vi "map construction.vi"() -> ()   [LabVIEW 2018]
uses:
  <vilib>/vision/NI_Vision_Development_Module.lvlib
panel:
  out "i":i32
  out "Image 7":T1(plugin-control)
  in  "Stop (F)":bool
  out "数值 2":dbl
  out "数值":dbl
  out "数组":sgl[](array[numeric])
  out "Objects":T2(array[cluster]) {"Aspect Ratio" format="%.2f"; "Orientation" format="%.2f"; "Area" format="%.2f"; "Object Center"."Y" format="%.2f"; "Object Center"."X" format="%.2f"}
  in  "Settings":T3={"Objects"=0, "Threshold"=128, "Reject Border"=FALSE, "Fill Holes"=FALSE, "Min Object Size"=TRUE, "Min Size"=5000, "Max Object Size"=FALSE, "Max Size"=100, "Show Search Area"=FALSE, "Show Center"=TRUE, "Show Bounding Box"=TRUE} {"Objects" items=["Bright Objects", "Dark Objects"]; "Threshold" min=1 max=999999999 step=1; "Max Size" min=1 max=999999999 step=1; "Min Size" min=1 max=999999999 step=1}
  out "Image 2":T1(plugin-control)
  in  "Range":cluster{"Lower value":sgl, "Upper value":sgl}={"Lower value"=0.0, "Upper value"=128.0} {"Upper value" format="%.2f"; "Lower value" format="%.2f"}
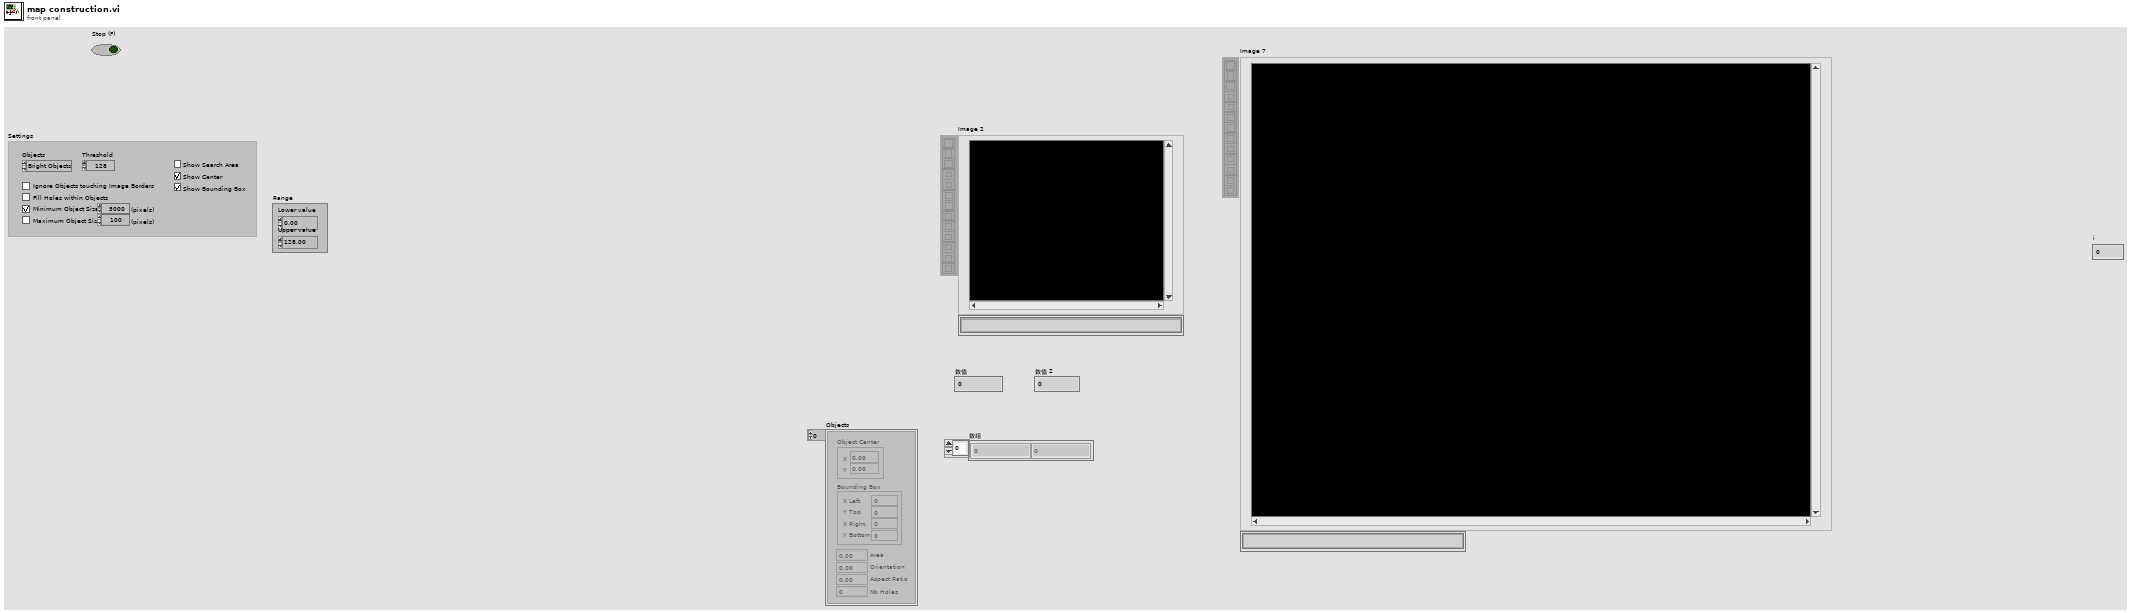
[diagram p1: front panel]
types:
  T1 = typedef "IMAQ Image.ctl" = refnum<image>
  T2 = cluster{"Object Center":cluster{"X":sgl, "Y":sgl}, "Bounding Box":cluster{"X Left":i32, "Y Top":i32, "X Right":i32, "Y Bottom":i32}, "Area":sgl, "Orientation":sgl, "Aspect Ratio":sgl, "Nb Holes":i32}[]
  T3 = cluster{"Objects":u16, "Threshold":i32, "Reject Border":bool, "Fill Holes":bool, "Min Object Size":bool, "Min Size":i32, "Max Object Size":bool, "Max Size":i32, "Show Search Area":bool, "Show Center":bool, "Show Bounding Box":bool}
  T4 = typedef "Image Type" = u32
  T5 = cluster{"Left":i32, "Top":i32, "Right":i32, "Bottom":i32}
  T6 = cluster{"Objects[0]":cluster{"Object Center":cluster{"X":sgl, "Y":sgl}, "Bounding Box":cluster{"X Left":i32, "Y Top":i32, "X Right":i32, "Y Bottom":i32}, "Area":sgl, "Orientation":sgl, "Aspect Ratio":sgl, "Nb Holes":i32}, "Objects[1]":cluster{"Object Center":cluster{"X":sgl, "Y":sgl}, "Bounding Box":cluster{"X Left":i32, "Y Top":i32, "X Right":i32, "Y Bottom":i32}, "Area":sgl, "Orientation":sgl, "Aspect Ratio":sgl, "Nb Holes":i32}, "Objects[2]":cluster{"Object Center":cluster{"X":sgl, "Y":sgl}, "Bounding Box":cluster{"X Left":i32, "Y Top":i32, "X Right":i32, "Y Bottom":i32}, "Area":sgl, "Orientation":sgl, "Aspect Ratio":sgl, "Nb Holes":i32}, "Objects[3]":cluster{"Object Center":cluster{"X":sgl, "Y":sgl}, "Bounding Box":cluster{"X Left":i32, "Y Top":i32, "X Right":i32, "Y Bottom":i32}, "Area":sgl, "Orientation":sgl, "Aspect Ratio":sgl, "Nb Holes":i32}, "Objects[4]":cluster{"Object Center":cluster{"X":sgl, "Y":sgl}, "Bounding Box":cluster{"X Left":i32, "Y Top":i32, "X Right":i32, "Y Bottom":i32}, "Area":sgl, "Orientation":sgl, "Aspect Ratio":sgl, "Nb Holes":i32}, "Objects[5]":cluster{"Object Center":cluster{"X":sgl, "Y":sgl}, "Bounding Box":cluster{"X Left":i32, "Y Top":i32, "X Right":i32, "Y Bottom":i32}, "Area":sgl, "Orientation":sgl, "Aspect Ratio":sgl, "Nb Holes":i32}, "Objects[6]":cluster{"Object Center":cluster{"X":sgl, "Y":sgl}, "Bounding Box":cluster{"X Left":i32, "Y Top":i32, "X Right":i32, "Y Bottom":i32}, "Area":sgl, "Orientation":sgl, "Aspect Ratio":sgl, "Nb Holes":i32}, "Objects[7]":cluster{"Object Center":cluster{"X":sgl, "Y":sgl}, "Bounding Box":cluster{"X Left":i32, "Y Top":i32, "X Right":i32, "Y Bottom":i32}, "Area":sgl, "Orientation":sgl, "Aspect Ratio":sgl, "Nb Holes":i32}, "Objects[8]":cluster{"Object Center":cluster{"X":sgl, "Y":sgl}, "Bounding Box":cluster{"X Left":i32, "Y Top":i32, "X Right":i32, "Y Bottom":i32}, "Area":sgl, "Orientation":sgl, "Aspect Ratio":sgl, "Nb Holes":i32}}
  T7 = cluster{"Object Center":cluster{"X":sgl, "Y":sgl}, "Bounding Box":cluster{"X Left":i32, "Y Top":i32, "X Right":i32, "Y Bottom":i32}, "Area":sgl, "Orientation":sgl, "Aspect Ratio":sgl, "Nb Holes":i32}
  T8 = cluster{"X Left":i32, "Y Top":i32, "X Right":i32, "Y Bottom":i32}
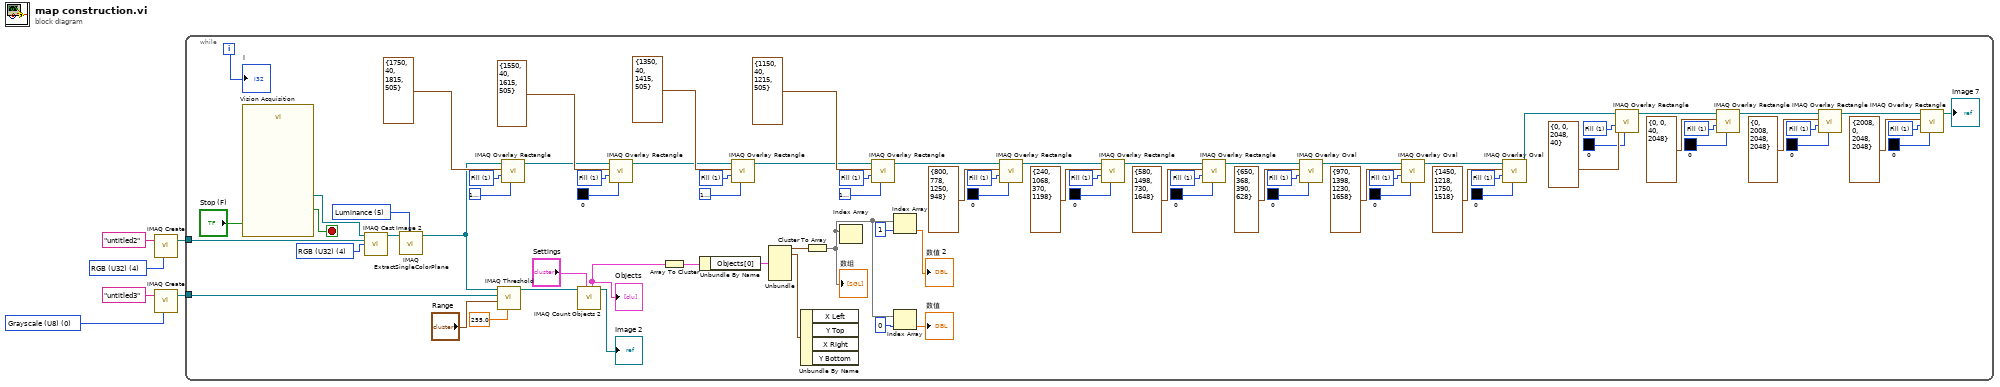
[diagram p0: block diagram]
diagram:
  w1 = T4 0 items=["Grayscale (U8)", "Grayscale (I16)", "Grayscale (SGL)", "Complex (CSG)", "RGB (U32)", "HSL (U32)", "RGB (U64)", "Grayscale (U16)"] ("Image Type")
  w4 = T4 4 items=["Grayscale (U8)", "Grayscale (I16)", "Grayscale (SGL)", "Complex (CSG)", "RGB (U32)", "HSL (U32)", "RGB (U64)", "Grayscale (U16)"] ("Image Type")
  n1 = call "IMAQ Create"("Image Name"="untitled2", "Image Type"=w4) -> ("New Image"=w5:T1)  [unwired: 3 in, 1 out]
  n2 = call "IMAQ Create"("Image Name"="untitled3", "Image Type"=w1) -> ("New Image"=w3:T1)  [unwired: 3 in, 1 out]
  n3 = while {
    tunnel: w5 -> [w87]
    tunnel: w3 -> [w83]
    i -> [w50]
    stop <- w72 stop-if-true
    w8 = u32 1 items=["Frame", "Fill", "Highlight"] ("Drawing Mode (Frame)")
    w11 = u32 1 items=["Frame", "Fill", "Highlight"] ("Drawing Mode (Frame)")
    w14 = u32 1 items=["Frame", "Fill", "Highlight"] ("Drawing Mode (Frame)")
    w17 = u32 1 items=["Frame", "Fill", "Highlight"] ("Drawing Mode (Frame)")
    w25 = u32 1 items=["Frame", "Fill"] ("Drawing Mode (Frame)")
    w28 = u32 1 items=["Frame", "Fill"] ("Drawing Mode (Frame)")
    w33 = u32 1 items=["Frame", "Fill"] ("Drawing Mode (Frame)")
    w46 = u32 1 items=["Frame", "Fill", "Highlight"] ("Drawing Mode (Frame)")
    w39 = u32 1 items=["Frame", "Fill"] ("Drawing Mode (Frame)")
    w49 = u32 1 items=["Frame", "Fill", "Highlight"] ("Drawing Mode (Frame)")
    w55 = u32 1 items=["Frame", "Fill", "Highlight"] ("Drawing Mode (Frame)")
    w58 = u32 1 items=["Frame", "Fill", "Highlight"] ("Drawing Mode (Frame)")
    w61 = u32 1 items=["Frame", "Fill", "Highlight"] ("Drawing Mode (Frame)")
    w64 = u32 1 items=["Frame", "Fill", "Highlight"] ("Drawing Mode (Frame)")
    w84 = T4 4 items=["Grayscale (U8)", "Grayscale (I16)", "Grayscale (SGL)", "Complex (CSG)", "RGB (U32)", "HSL (U32)", "RGB (U64)", "Grayscale (U16)"] ("Image Type")
    w86 = 5 items=["Red", "Green", "Blue", "Hue", "Saturation", "Luminance", "Value", "Intensity"] ("Color Plane")
    n4 = call "Vision Acquisition"("Stop (F)"="Stop (F)") -> ("Image Out"=w67:T1, "Stopped"=w72:bool)  [unwired: 24 in, 1 out]
    n5 = call "IMAQ Cast Image 2"("Image Src"=w67, "Image Dst"=w87, "Image Type"=w84) -> ("Image Dst Out"=w85:T1)  [unwired: 11 in, 1 out]
    n6 = call "IMAQ ExtractSingleColorPlane"("Color Plane"=w86, "Image Src"=w85) -> ("Image Dst Out"=w37:T1)  [unwired: 8 in, 1 out]
    n7 = call "IMAQ Threshold"("Replace Value"=sgl 255.0, "Range"="Range", "Image Dst"=w83, "Image Src"=w37) -> ("Image Dst Out"=w65:T1)  [unwired: 6 in, 1 out]
    n8 = call "IMAQ Overlay Rectangle"("Color"=u32 16777222, "Drawing Mode (Frame)"=w58, "Rectangle"=T5 {"Left"=1750, "Top"=40, "Right"=1815, "Bottom"=505}, "Image"=w37) -> ("Image Out"=w36:T1)  [unwired: 6 in, 1 out]
    n9 = call "IMAQ Count Objects 2"("Settings"="Settings", "Image"=w65) -> ("Image Out"=→"Image 2":T1, "Objects"=w79:T2)  [unwired: 5 in, 3 out]
    "Objects" <- w79
    n10 = call "IMAQ Overlay Rectangle"("Color"=u32 0, "Drawing Mode (Frame)"=w55, "Rectangle"=T5 {"Left"=1550, "Top"=40, "Right"=1615, "Bottom"=505}, "Image"=w36) -> ("Image Out"=w52:T1)  [unwired: 6 in, 1 out]
    n11 = Array To Cluster(array=w79) -> (cluster=w78:T6)
    n12 = Unbundle By Name(w78) -> ("Objects[0]"=w77:T7)
    n13 = call "IMAQ Overlay Rectangle"("Color"=u32 16777222, "Drawing Mode (Frame)"=w61, "Rectangle"=T5 {"Left"=1350, "Top"=40, "Right"=1415, "Bottom"=505}, "Image"=w52) -> ("Image Out"=w51:T1)  [unwired: 6 in, 1 out]
    n14 = Unbundle(w77) -> ("Object Center"=w76:cluster{"X":sgl, "Y":sgl}, "Bounding Box"=w66:T8)  [unwired: 4 out]
    n15 = Unbundle By Name(w66) -> ()  [unwired: 4 out]
    n16 = Cluster To Array(cluster=w76) -> (array=w74:sgl[])
    "数组" <- w74
    n17 = Index Array(array=w74) -> ()  [unwired: 1 in, 1 out]
    n18 = call "IMAQ Overlay Rectangle"("Color"=u32 16777222, "Drawing Mode (Frame)"=w64, "Rectangle"=T5 {"Left"=1150, "Top"=40, "Right"=1215, "Bottom"=505}, "Image"=w51) -> ("Image Out"=w38:T1)  [unwired: 6 in, 1 out]
    n19 = Index Array(array=w74, index=1 ("索引")) -> (element=→"数值 2":sgl)
    n20 = Index Array(array=w74, index=0 ("索引")) -> (element=→"数值":sgl)
    n21 = call "IMAQ Overlay Rectangle"("Color"=u32 0, "Drawing Mode (Frame)"=w49, "Rectangle"=T5 {"Left"=800, "Top"=778, "Right"=1250, "Bottom"=948}, "Image"=w38) -> ("Image Out"=w42:T1)  [unwired: 6 in, 1 out]
    n22 = call "IMAQ Overlay Rectangle"("Color"=u32 0, "Drawing Mode (Frame)"=w39, "Rectangle"=T5 {"Left"=240, "Top"=1068, "Right"=370, "Bottom"=1198}, "Image"=w42) -> ("Image Out"=w43:T1)  [unwired: 6 in, 1 out]
    n23 = call "IMAQ Overlay Rectangle"("Color"=u32 0, "Drawing Mode (Frame)"=w46, "Rectangle"=T5 {"Left"=580, "Top"=1498, "Right"=730, "Bottom"=1648}, "Image"=w43) -> ("Image Out"=w35:T1)  [unwired: 6 in, 1 out]
    n24 = call "IMAQ Overlay Oval"("Color"=u32 0, "Drawing Mode (Frame)"=w33, "Bounding Rectangle"=T5 {"Left"=650, "Top"=368, "Right"=390, "Bottom"=628}, "Image"=w35) -> ("Image Out"=w30:T1)  [unwired: 6 in, 1 out]
    n25 = call "IMAQ Overlay Oval"("Color"=u32 0, "Drawing Mode (Frame)"=w28, "Bounding Rectangle"=T5 {"Left"=970, "Top"=1398, "Right"=1230, "Bottom"=1658}, "Image"=w30) -> ("Image Out"=w31:T1)  [unwired: 6 in, 1 out]
    n26 = call "IMAQ Overlay Oval"("Color"=u32 0, "Drawing Mode (Frame)"=w25, "Bounding Rectangle"=T5 {"Left"=1450, "Top"=1218, "Right"=1750, "Bottom"=1518}, "Image"=w31) -> ("Image Out"=w23:T1)  [unwired: 6 in, 1 out]
    n27 = call "IMAQ Overlay Rectangle"("Color"=u32 0, "Drawing Mode (Frame)"=w17, "Rectangle"=T5 {"Left"=0, "Top"=0, "Right"=2048, "Bottom"=40}, "Image"=w23) -> ("Image Out"=w22:T1)  [unwired: 6 in, 1 out]
    n28 = call "IMAQ Overlay Rectangle"("Color"=u32 0, "Drawing Mode (Frame)"=w14, "Rectangle"=T5 {"Left"=0, "Top"=0, "Right"=40, "Bottom"=2048}, "Image"=w22) -> ("Image Out"=w21:T1)  [unwired: 6 in, 1 out]
    n29 = call "IMAQ Overlay Rectangle"("Color"=u32 0, "Drawing Mode (Frame)"=w11, "Rectangle"=T5 {"Left"=0, "Top"=2008, "Right"=2048, "Bottom"=2048}, "Image"=w21) -> ("Image Out"=w20:T1)  [unwired: 6 in, 1 out]
    n30 = call "IMAQ Overlay Rectangle"("Color"=u32 0, "Drawing Mode (Frame)"=w8, "Rectangle"=T5 {"Left"=2008, "Top"=0, "Right"=2048, "Bottom"=2048}, "Image"=w20) -> ("Image Out"=→"Image 7":T1)  [unwired: 6 in, 1 out]
    "i" <- w50
  }
